vi "Configure Current List.vi"(8 "error in (no error)":errorcluster, 9 "Dwell Points":dbl[](array[numeric]), 10 "Current Points":dbl[](array[numeric]), 11 "VISA resource name":refnum<visa-resource-name>) -> (0 "error out":errorcluster, 3 "VISA resource name out":refnum<visa-resource-name>)   [LabVIEW 2019, in "Agilent N7976A.lvlib"]
doc: "Configures the current and dwell lists when current priority mode."
uses:
  <instrlib>/Agilent N7976A/Agilent N7976A.lvlib
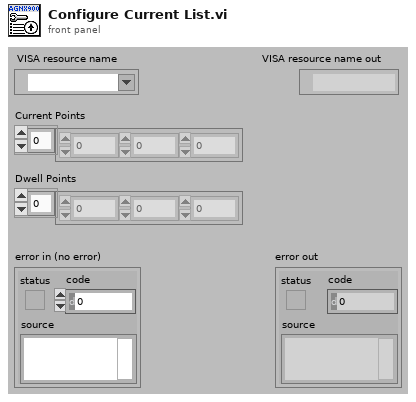
[diagram p1: front panel]
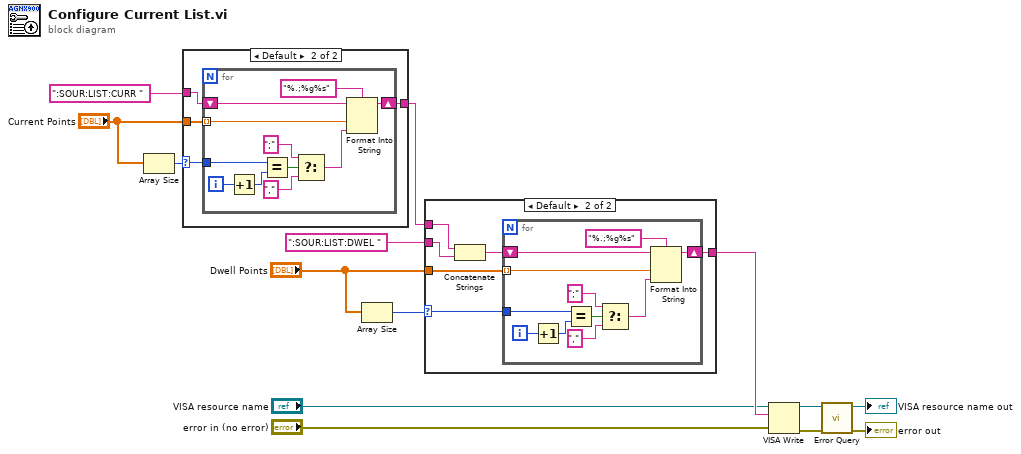
[diagram p0: block diagram]
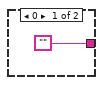
[diagram p2: hidden frame]
diagram:
  n1 = Array Size(array="Current Points") -> (size(s)=w13:i32)
  n2 = case shown="Default" w13 {
    selector: w13 -> [_ w17]
    tunnel: "Current Points" -> [_ w18]
    tunnel: ":SOUR:LIST:CURR " -> [_ w19]
    tunnel: ["" w16] -> w14
    frame 0 {
    }
    frame Default {
      n3 = for {
        shift-right: [w21] -> w16
        shift-left: w19 -> [w24]
        tunnel: w18 -> [w23] mode=indexing
        tunnel: w17 -> [w28]
        i -> [w30]
        n4 = Increment(x=w30) -> (x+1=w29:i32)
        n5 = Equal?(x=w28, y=w29) -> (x = y?=w27:bool)
        n6 = Select(t=";", s=w27, f="," ("t")) -> (s? t:f=w22:string)
        n7 = Format Into String(format string="%.;%g%s", initial string=w24, w23, w22) -> (resulting string=w21:string)  [unwired: 1 in, 1 out]
      }
    }
  }
  n8 = Array Size(array="Dwell Points") -> (size(s)=w1:i32)
  n9 = case shown="Default" w1 {
    selector: w1 -> [_ w36]
    tunnel: "Dwell Points" -> [_ w37]
    tunnel: ":SOUR:LIST:DWEL " -> [_ w33]
    tunnel: [w31 w35] -> w8
    tunnel: w14 -> [w31 w34]
    frame 0 {
    }
    frame Default {
      n10 = Concatenate Strings(w34, w33) -> (w32:string)
      n11 = for {
        shift-right: [w39] -> w35
        shift-left: w32 -> [w42]
        tunnel: w37 -> [w41] mode=indexing
        tunnel: w36 -> [w46]
        i -> [w48]
        n12 = Increment(x=w48) -> (x+1=w47:i32)
        n13 = Equal?(x=w46, y=w47) -> (x = y?=w45:bool)
        n14 = Select(t=";", s=w45, f="," ("t")) -> (s? t:f=w40:string)
        n15 = Format Into String(format string="%.;%g%s", initial string=w42, w41, w40) -> (resulting string=w39:string)  [unwired: 1 in, 1 out]
      }
    }
  }
  n16 = VISA Write(VISA resource name="VISA resource name", write buffer=w8, error in (no error)="error in (no error)") -> (VISA resource name out=w7:refnum<visa-resource-name>, error out=w6:errorcluster)  [unwired: 1 out]
  n17 = call <instrlib>:"Error Query.vi"("error in (no error)"=w6, "VISA resource name"=w7) -> ("error out"=→"error out":errorcluster, "VISA resource name out"=→"VISA resource name out":refnum<visa-resource-name>)  [unwired: 6 in, 2 out]
